vi "n set firstpulse killer list.vi"(8 "error in (no error)":errorcluster, 10 "fpk":u16, 11 "n":u16) -> (0 "error out":errorcluster)   [LabVIEW 2015, in "SCANalone4x64.lvlib"]
doc: "__declspec(dllimport) void __stdcall n_set_firstpulse_killer_list(unsigned short n, unsigned short fpk);"
uses:
  <userlib>/SCANalone4x64/SCANalone4x64.lvlib
  <userlib>/SCANalone4x64/SCANalone4x64.dll
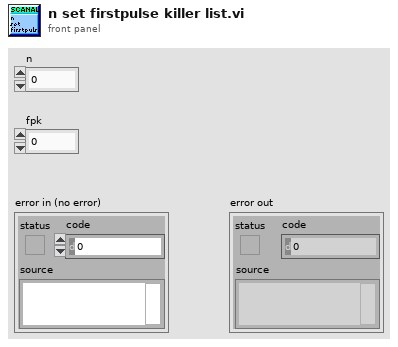
[diagram p1: front panel]
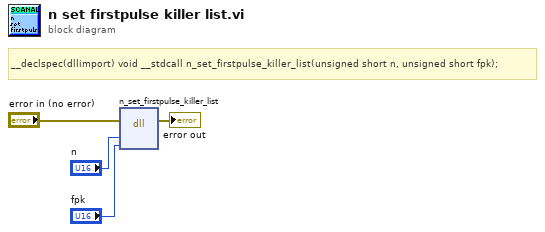
[diagram p0: block diagram]
diagram:
  # "__declspec(dllimport) void __stdcall n_set_firstpulse_killer_list(unsigned short n, unsigned short fpk);"
  n1 = dll-call lib="C:/Program Files/National Instruments/LabVIEW 2015/user.lib/SCANalone4x64/SCANalone4x64.*" fn="n_set_firstpulse_killer_list"(error in="error in (no error)", "n"="n", "fpk"="fpk") -> (error out=→"error out":errorcluster)  [unwired: 5 in, 1 out]
